vi "Initialize.vi"(8 "error in":errorcluster, 11 "Reversi in":refnum<class "Reversi.lvclass">) -> (0 "error out":errorcluster, 3 "Reversi out":refnum<class "Reversi.lvclass">)   [LabVIEW 2020, in "Reversi.lvlib" / "Reversi.lvclass"]
uses:
  Reversi.lvclass
  Space Ring.ctl
  Space Cluster.ctl
  Space Coordinates.ctl
  Reversi.lvclass/Reversi.ctl
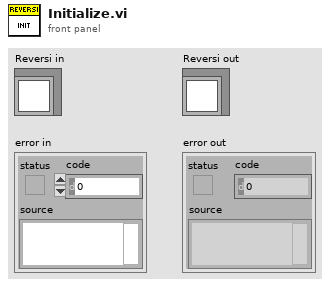
[diagram p1: front panel]
types:
  T1 = typedef "Reversi.lvlib/Reversi.lvclass/Space Cluster.ctl" = cluster{"Coordinates":T2, "Ring":T3}
  T2 = typedef "Reversi.lvlib/Reversi.lvclass/Space Coordinates.ctl" = cluster{"Row":i32, "Column":i32}
  T3 = typedef "Reversi.lvlib/Reversi.lvclass/Space Ring.ctl" = u16
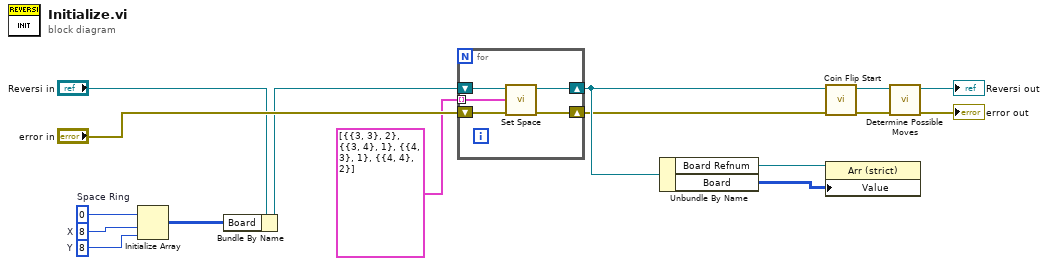
[diagram p0: block diagram]
diagram:
  w9 = T3 0  # Space Ring
  w11 = 8  # Y
  w12 = 8  # X
  n1 = Initialize Array(w9, w12, w11) -> (w5:T3[][])
  n2 = Bundle By Name(cluster="Reversi in", "Board"=w5) -> (w10:refnum<class "Reversi.lvclass">)
  n3 = for {
    shift-right: [w18] -> w2
    shift-left: w10 -> [w19]
    shift-right: [w20] -> w1
    shift-left: "error in" -> [w21]
    tunnel: T1[] [{"Coordinates"={"Row"=3, "Column"=3}, "Ring"=2}, {"Coordinates"={"Row"=3, "Column"=4}, "Ring"=1}, {"Coordinates"={"Row"=4, "Column"=3}, "Ring"=1}, {"Coordinates"={"Row"=4, "Column"=4}, "Ring"=2}] -> [w17] mode=indexing
    n4 = call "Set Space.vi"("error in (no error)"=w21, "Space"=w17, "Reversi in"=w19) -> ("error out"=w20:errorcluster, "Reversi out"=w18:refnum<class "Reversi.lvclass">)  [unwired: 7 in]
  }
  n5 = Unbundle By Name(w2) -> ("Board Refnum"=w3:refnum<vi>, "Board"=w4:T3[][])
  n6 = call "Coin Flip Start.vi"("error in (no error)"=w1, "Reversi in"=w2) -> ("error out"=w16:errorcluster, "Reversi out"=w7:refnum<class "Reversi.lvclass">)  [unwired: 8 in]
  n7 = property class="Arr (strict)"(reference=w3, "Value"=w4) -> ()  [unwired: 1 in, 2 out]
  n8 = call "Determine Possible Moves.vi"("error in (no error)"=w16, "Reversi in"=w7) -> ("error out"=→"error out":errorcluster, "Reversi out"=→"Reversi out":refnum<class "Reversi.lvclass">)  [unwired: 8 in]
